vi "Start.vi"() -> ()   [LabVIEW 2014]
panel:
  out "Start Balancing":bool
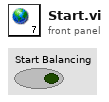
[diagram p1: front panel]
diagram:
